vi "Save Frecuency.vi"(8 "error in (no error)":errorcluster, 11 "frecuency":i32) -> (0 "error out":errorcluster)   [LabVIEW 2020, in "DataBase.lvlib"]
uses:
  DataBase.lvlib
  <vilib>/drjdpowell/SQLite Library/SQL Connection/Open (path).vi
  <vilib>/drjdpowell/SQLite Library/SQL Connection/Open (string).vi
  <vilib>/AdvancedString/Path To Command Line String.vi
  <vilib>/drjdpowell/SQLite Library/SQL Connection/Execute SQL (No results).vi
  <vilib>/drjdpowell/SQLite Library/SQL Connection/Connection.lvclass
  <vilib>/drjdpowell/SQLite Library/SQLite.lvlib
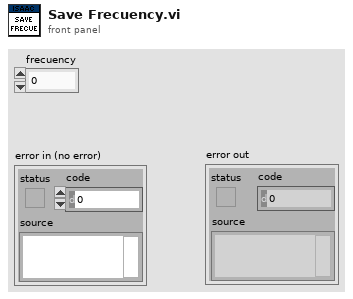
[diagram p1: front panel]
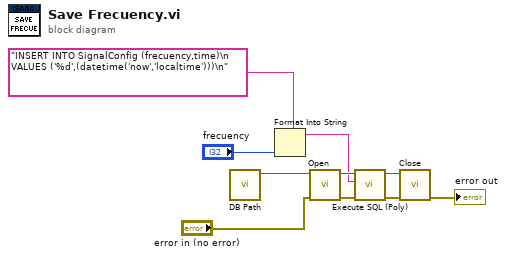
[diagram p0: block diagram]
diagram:
  n1 = call "DB Path.vi"() -> ("appended path"=w4:path)  [unwired: 11 in]
  n2 = Format Into String(format string="INSERT INTO SignalConfig (frecuency,time)\n VALUES ('%d',(datetime('now','localtime')))\n", "frecuency") -> (resulting string=w6:string)  [unwired: 2 in, 1 out]
  n3 = call-poly <vilib>:"Open.vi"("error in (no error)"="error in (no error)", "db file"=w4) -> ("error out"=w10:errorcluster, "SQLite Connection"=w9:refnum<class "Connection.lvclass">)  [unwired: 8 in]
  n4 = call-poly <vilib>:"Execute SQL (Poly).vi"("error in (no error)"=w10, "SQL"=w6, "SQLite Connection in"=w9) -> ("error out"=w8:errorcluster, "SQLite Connection"=w7:refnum<class "Connection.lvclass">)  [unwired: 7 in]
  n5 = call-dynamic "Close.vi"("error in (no error)"=w8, "SQLite Connection in"=w7) -> ("error out"=→"error out":errorcluster)  [unwired: 9 in]
